vi "Initialize Front Panel.vi"(8 "error in (no error)":errorcluster, 11 "IMediatorBusMonitor in":refnum<class "IMediatorBusMonitor.lvclass">) -> (0 "error out":errorcluster, 3 "IMediatorBusMonitor out":refnum<class "IMediatorBusMonitor.lvclass">)   [LabVIEW 2015, in "IMediator.lvlib" / "IMediatorBusMonitor.lvclass"]
doc: "<License>\nCopyright © 2017 Composed Systems, LLC | All rights reserved\nwww.composed.io\n\nAuthor: Ethan Stern <ethan.stern@composed.io>\n\nThis software is provided \"AS IS\" WITHOUT WARRANTIES, either express or implied, AND IS FOR EDUCATIONAL PURPOSES ONLY.\n</License>"
uses:
  IMediatorBusMonitor.lvclass
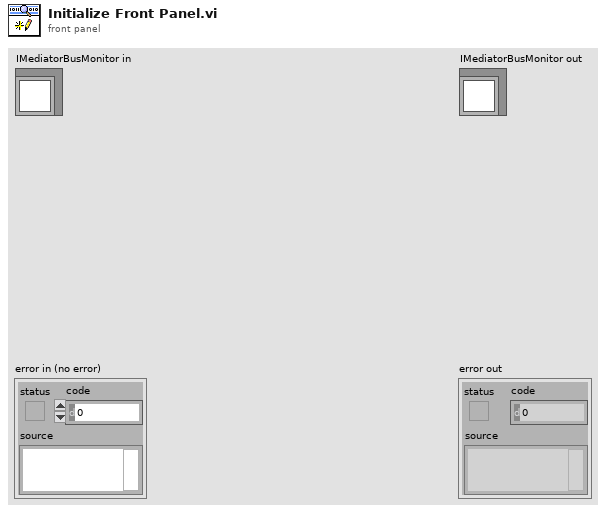
[diagram p1: front panel]
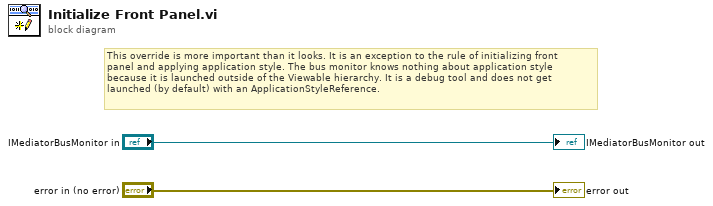
[diagram p0: block diagram]
diagram:
  # "This override is more important than it looks. It is an exception to the rule of initializing front\npanel and applying application style. The bus monitor knows nothing about application style\nbecause it is launched outside of the Viewable hierarchy. It is a debug tool and does not get\nlaunched (by default) with an ApplicationStyleReference."
  "error out" <- "error in (no error)"
  "IMediatorBusMonitor out" <- "IMediatorBusMonitor in"
